vi "String To 1D U32.vi"(7 "Delimiter":string=",", 10 "String In":string) -> (2 "1D U32 Out":u32[](array[numeric]))   [LabVIEW 2024]
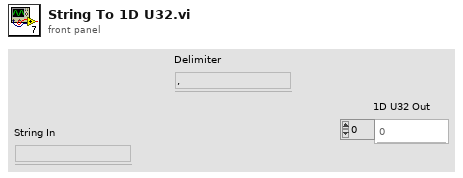
[diagram p1: front panel]
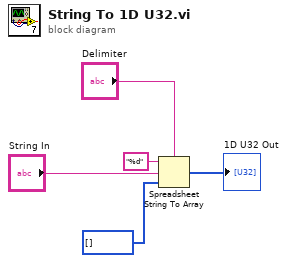
[diagram p0: block diagram]
diagram:
  n1 = Spreadsheet String To Array(delimiter (Tab)="Delimiter", format string="%d", spreadsheet string="String In", array type (2D Dbl)=u32[] []) -> (array=→"1D U32 Out":u32[])
